vi "createILCDAC.vi"(8 "error in (no error)":errorcluster, 9 "Channel":u8=1 min=1 max=4, 10 "ILC":refnum<class "ILC.lvclass">, 11 "IILCDACFactory in":refnum<class "IILCDACFactory.lvclass">) -> (0 "error out":errorcluster, 2 "ILCDAC":refnum<class "IILCDAC.lvclass">, 3 "IILCDACFactory out":refnum<class "IILCDACFactory.lvclass">)   [LabVIEW 2015, in "IILCDACFactory.lvclass"]
uses:
  IILCDACFactory.lvclass
  <userlib>/Common/ILC/ILC/ILC.lvclass
  ILCDAC/IILCDAC/IILCDAC.lvclass
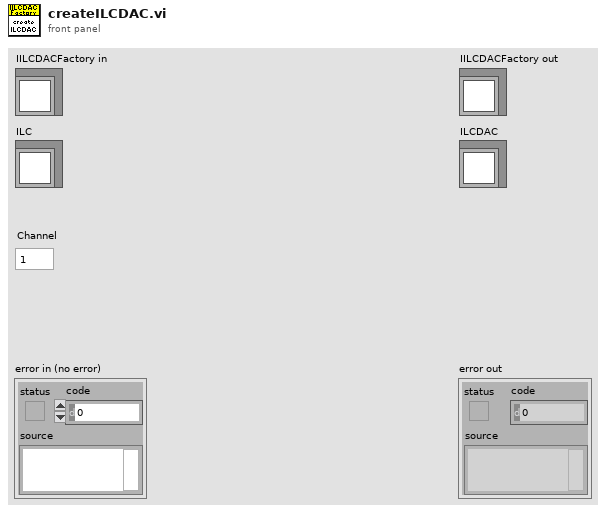
[diagram p1: front panel]
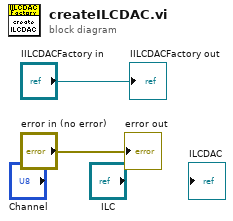
[diagram p0: block diagram]
diagram:
  "error out" <- "error in (no error)"
  "IILCDACFactory out" <- "IILCDACFactory in"
